vi "ScaleWaveForm.vi"(8 "error in (no error)":errorcluster, 11 "Waveform":waveform(sgl)) -> (0 "error out":errorcluster, 3 "Scaled Waveform":waveform(sgl))   [LabVIEW 2015]
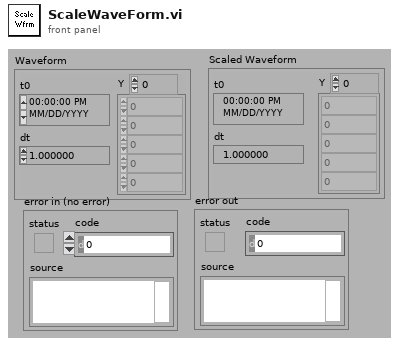
[diagram p1: front panel]
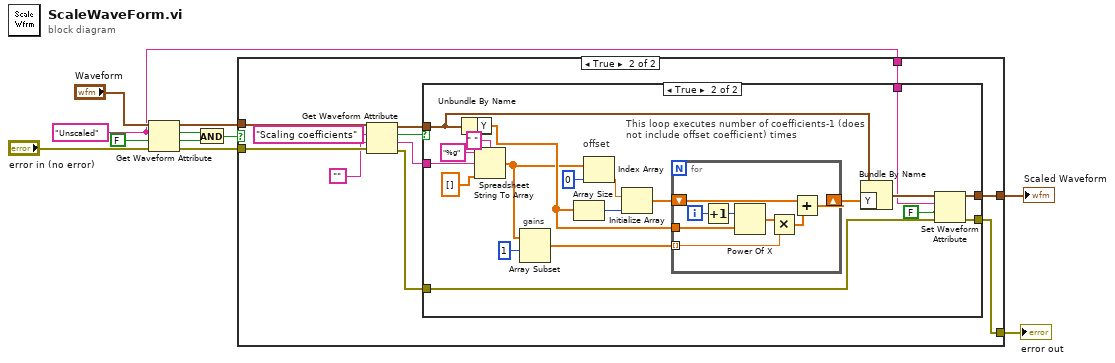
[diagram p0: block diagram]
diagram:
  w1 = "Unscaled"
  n1 = Get Waveform Attribute(4:"error in (no error)", 5:FALSE, 6:w1, 7:"Waveform") -> (0:w6:errorcluster, 1:w8:bool, 2:w7:bool, 3:w5:waveform(sgl))
  n2 = And(x=w7, y=w8) -> (x .and. y?=w4:bool)
  n3 = case shown="True" w4 {
    tunnel: w6 -> [w13 w24]
    tunnel: w5 -> [w12 w23]
    tunnel: [w12 w17] -> w3
    tunnel: [w13 w14] -> w2
    tunnel: w1 -> [_ w15]
    frame False {
    }
    frame True {
      n4 = Get Waveform Attribute(4:w24, 5:"", 6:"Scaling coefficients" ("name"), 7:w23) -> (0:w16:errorcluster, 1:w20:string, 2:w19:bool, 3:w18:waveform(sgl))
      n5 = case shown="True" w19 {
        tunnel: w20 -> [_ w45]
        tunnel: w18 -> [w26 w36]
        tunnel: [w26 w32] -> w17
        tunnel: w16 -> [w25 w29]
        tunnel: w15 -> [_ w31]
        tunnel: [w25 w28] -> w14
        frame False {
        }
        frame True {
          # "This loop executes number of coefficients-1 (does\nnot include offset coefficient) times"
          # "offset"
          # "gains"
          n6 = Unbundle By Name(w36) -> ("Y"=w40:sgl[])
          n7 = Spreadsheet String To Array(delimiter (Tab)=" ", format string="%g", spreadsheet string=w45, array type (2D Dbl)=dbl[] []) -> (array=w37:dbl[])
          n8 = Array Subset(array=w37, index=1) -> (w44:dbl[])  [unwired: 1 in]
          n9 = Array Size(array=w40) -> (size(s)=w41:i32)
          n10 = Index Array(array=w37, index=0) -> (element=w43:dbl)
          n11 = Initialize Array(w43, w41) -> (w42:dbl[])
          n12 = for {
            shift-right: [w52] -> w35
            shift-left: w42 -> [w47]
            tunnel: w44 -> [w53] mode=indexing
            tunnel: w40 -> [w51]
            i -> [w54]
            n13 = Increment(x=w54) -> (x+1=w50:i32)
            n14 = Power Of X(1:w51, 2:w50) -> (0:w49:sgl[])
            n15 = Multiply(x=w49, y=w53) -> (x*y=w48:dbl[])
            n16 = Add(x=w47, y=w48) -> (x+y=w52:dbl[])
          }
          n17 = Bundle By Name(cluster=w36, "Y"=w35) -> (w33:waveform(sgl))
          n18 = Set Waveform Attribute(4:w29, 5:FALSE, 6:w31, 7:w33) -> (0:w28:errorcluster, 3:w32:waveform(sgl))  [unwired: 1 out]
        }
      }
    }
  }
  "Scaled Waveform" <- w3
  "error out" <- w2
